vi "FTW-SQLite-CloseConnection.vi"(0 "SQLite Connection":refnum<data-value>, 11 "error in":errorcluster) -> (15 "error out":errorcluster)   [LabVIEW 2015]
uses:
  core/FTW-SQLite-Core-Structure.ctl
panel:
  # "Inputs"
  # "Outputs"
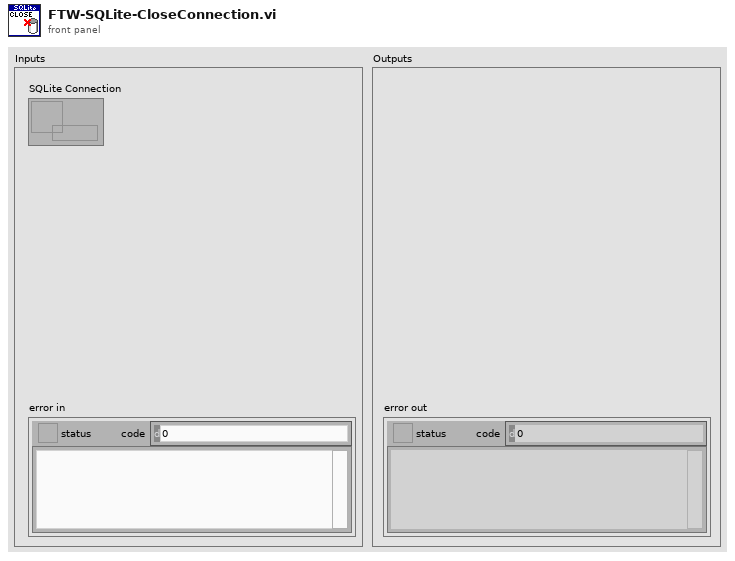
[diagram p1: front panel]
types:
  T1 = typedef "FTW-SQLite-Core-Structure.ctl" = cluster{"Connection":u64}
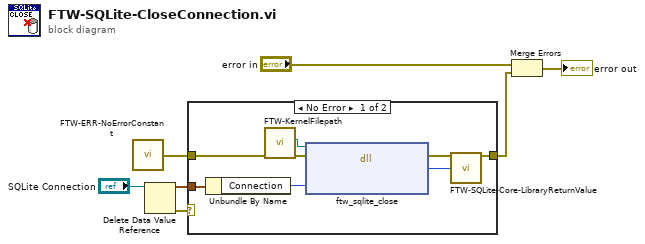
[diagram p0: block diagram]
diagram:
  n1 = call "FTW-ERR-NoErrorConstant.vi"() -> ("no error"=w1:errorcluster)
  n2 = Delete Data Value Reference(data value reference="SQLite Connection") -> (data value=w3:T1, error out=w2:errorcluster)  [unwired: 1 in]
  n3 = case shown="No Error" w2 {
    tunnel: [w13 w16] -> w6
    tunnel: w3 -> [w12 _]
    tunnel: w1 -> [w10 w16]
    frame No Error {
      n4 = Unbundle By Name(w12) -> ("Connection"=w11:u64)
      n5 = call "FTW-KernelFilepath.vi"("error in"=w10) -> ("error out"=w9:errorcluster, "Library Filepath"=w8:path)  [unwired: 8 in, 1 out]
      n6 = dll-call lib="?" fn="ftw_sqlite_close"(path in=w8, error in=w9, "Connection Handle"=w11) -> (error out=w15:errorcluster, "Return Value"=w14:i32)  [unwired: 2 in, 1 out]
      n7 = call "FTW-SQLite-Core-LibraryReturnValue.vi"("error in"=w15, "Return Value"=w14) -> ("error out"=w13:errorcluster)  [unwired: 13 in]
    }
    frame Error {
    }
  }
  n8 = Merge Errors("error in", w6) -> (→"error out":errorcluster)
